vi "simple_cache.vi"(1 "refresh":bool, 2 "new_val":fxp<+/-,32,16>) -> (0 "$_val":fxp<+/-,32,16>)   [LabVIEW 2018]
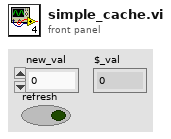
[diagram p1: front panel]
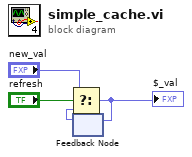
[diagram p0: block diagram]
diagram:
  n1 = feedback #1() -> (w1:fxp<+/-,32,16>)  [unwired: 1 in]
  n2 = Select(t="new_val", s="refresh", f=w1) -> (s? t:f=w2:fxp<+/-,32,16>)
  "$_val" <- w2
  n3 = feedback-in #1(w2) -> ()
